vi "Panel.vi"(6 "Fiber Auto Collimation state data":refnum<class "Fiber Auto Collimation state data.lvclass">, 7 "Station config":refnum<class "Station config.lvclass">, 8 "error in":errorcluster, 11 "Fiber Auto Collimation main panel in":refnum<class "Fiber Auto Collimation main panel.lvclass">) -> (0 "error out":errorcluster, 3 "Fiber Auto Collimation main panel out":refnum<class "Fiber Auto Collimation main panel.lvclass">)   [LabVIEW 2018, in "Fiber Auto Collimation main panel.lvclass"]
doc: "The main panel of the station template when it's created. Adjust as needed!"
uses:
  Fiber Auto Collimation main panel.lvclass
  State data/BV Data.ctl
  C:/LabVIEW code/Fiber Auto Collimation/Source/Panels/Fiber Auto Collimation panel.lvclass
  State data/Fiber Auto Collimation state data.lvclass
  <userlib>/Recipe/Station Config/Station config.lvclass
  C:/Program Files (x86)/National Instruments/LabVIEW 2018/user.lib/Recipe/nLight Recipe/nLight Recipe.lvclass
  State data/Permission levels.ctl
  State data/Tracked state data.ctl
  State data/Instrument list.ctl
  State data/Fiber Auto Collimation state data.lvclass/Fiber Auto Collimation state data.ctl
  State data/String keys.ctl
  <userlib>/Recipe/Station Config/Station config.lvclass/Station config.ctl
  403c9101-8a94-4915-b1d2-c2bcb50c0ac3.vi
  4715e2b4-8d0b-45f9-9f48-fce3cbe10ad4.vi
  ee343da0-43c2-4897-a8b1-c706a9c51c79.vi
  88e119a9-a23e-4267-b647-8cd8f19a308b.vi
  457d34be-29b3-4e5e-81a2-a964ebca1608.vi
  94bc7fe1-a039-41b1-a3da-682790e1e5e6.vi
  5b4d40ab-973c-4ebc-87e6-d7e06bf2d1ec.vi
  373ea118-2318-4414-a1df-ab0a70bb7f1d.vi
  0939716d-f432-4146-8606-eb2c000bf93c.vi
  14963872-09c7-484d-8f8b-814a5689ce7f.vi
  226fbdc5-8833-4035-85a3-cb53d1a6b5a4.vi
  403c9101-8a94-4915-b1d2-c2bcb50c0ac3.vi/f33612d2-cbd2-4a12-8b29-77b7af87b990.vi
  88e119a9-a23e-4267-b647-8cd8f19a308b.vi/82f232c0-e180-498c-b36d-e812967a056b.vi
  References/Obtain control updates queue.vi
  Misc SubVIs/Get control name.vi
  <userlib>/nLight Error Handling/Merge errors no loss.vi
  <userlib>/nLight Error Handling/Replace string to enum conversion error.vi
  <userlib>/nLight Error Handling/Insert error no loss.vi
  <instrlib>/nLight Instruments/Monitor/Read History array.vi
  <vilib>/Utility/Data Type/Get Type Information.vi
  <userlib>/nLight Error Handling/Log any errors.vi
  <userlib>/Recipe/Test Recipe classes/Test Recipe.lvclass
  <instrlib>/nLight Instruments/nLight Instrument/nLight Instrument.lvclass
  <instrlib>/nLight Instruments/Monitor/Monitor.lvclass
  a23b397d-d5c1-4275-a046-494f1c6e56ee.vi
  <userlib>/Recipe/nLight Recipe/nLight Recipe.lvclass
  <userlib>/nEQdb/Test Data classes/Test Data.lvclass
  References/Fiber Auto Collimation References.lvclass
  Fiber Auto Collimation panel.lvclass
panel:
  in  "Defect detection":bool
  in  "Save Data":bool
  in  "SN selection":string(combo)
  in  "Step Size 6":bool
  in  "Step Size 5":bool
  in  "Step Size 4":bool
  in  "Step Size 3":bool
  in  "Step Size 2":bool
  in  "Step Size 1":bool
  in  "Spot detection":bool
  in  "Collimation":bool
  in  "Manual Mode":bool
  in  "Auto Mode":bool
  in  "Operator":string
  in  "Fiber Ass PN":string
  in  "SN-5":string
  in  "SN-4":string
  in  "SN-3":string
  in  "SN-2":string
  in  "SN-1":string
  in  "MOM Lot-2":string caption="MOM Lot"
  out "Measurement Report":string
  out "Collimation Image":T1(plugin-control)
  out "BV Data":T2={"Centroid X[um]"=nan, "Centroid Y[um]"=nan, "PeakResp.[%]"=nan, "Knife Edge X[mm]"=nan, "Knife Edge Y[mm]"=nan, "Circularity"=nan, "Collimation Result"=FALSE}
  in  "Cancel Test":bool
  in  "Start Test":bool
  in  "Enter MOM Lot":bool
  out "Test status":string
  out "MOM Lot":string
  out "Recipe Name":string
  out "Test in progress":bool
  out "DUT Serial":string
  out "Current Position[mm]":dbl
  in  "Home":bool
  in  "Down":bool
  in  "Up":bool
  out "Distance":dbl[unit] caption="Current step size" min=-0.001 max=0.025 step=0.001
  in  "Remote stop config panel":bool
  in  "Open and embed config panel":bool
  in  "Open config panel":bool
  out "Station information":string="Software name: \nSoftware version:\nSite: \nEnvironment: \nNEQdb Station number: \nMOM Equipment ID: "
  out "Monitored Watt indicator":dbl[unit]
  out "Fake LIV graph - Should be deleted later":T3(graph)
  out "Currently running state":string
  out "Username":string
  out "Permission level":T4
  out "Monitor Status":string
  # "INTRODUCE"
  # "Adjustment"
  # "Step size:"
  # "未连接MOM系统\n暂不使用"
  # "Settings"
  # "For the demo Monitor code.  Delete if not using Monitors at all.  If using Monitors, it may be useful to leave these as example code until after you implement your own monitors.  If so, you should probably hide both controls instead."
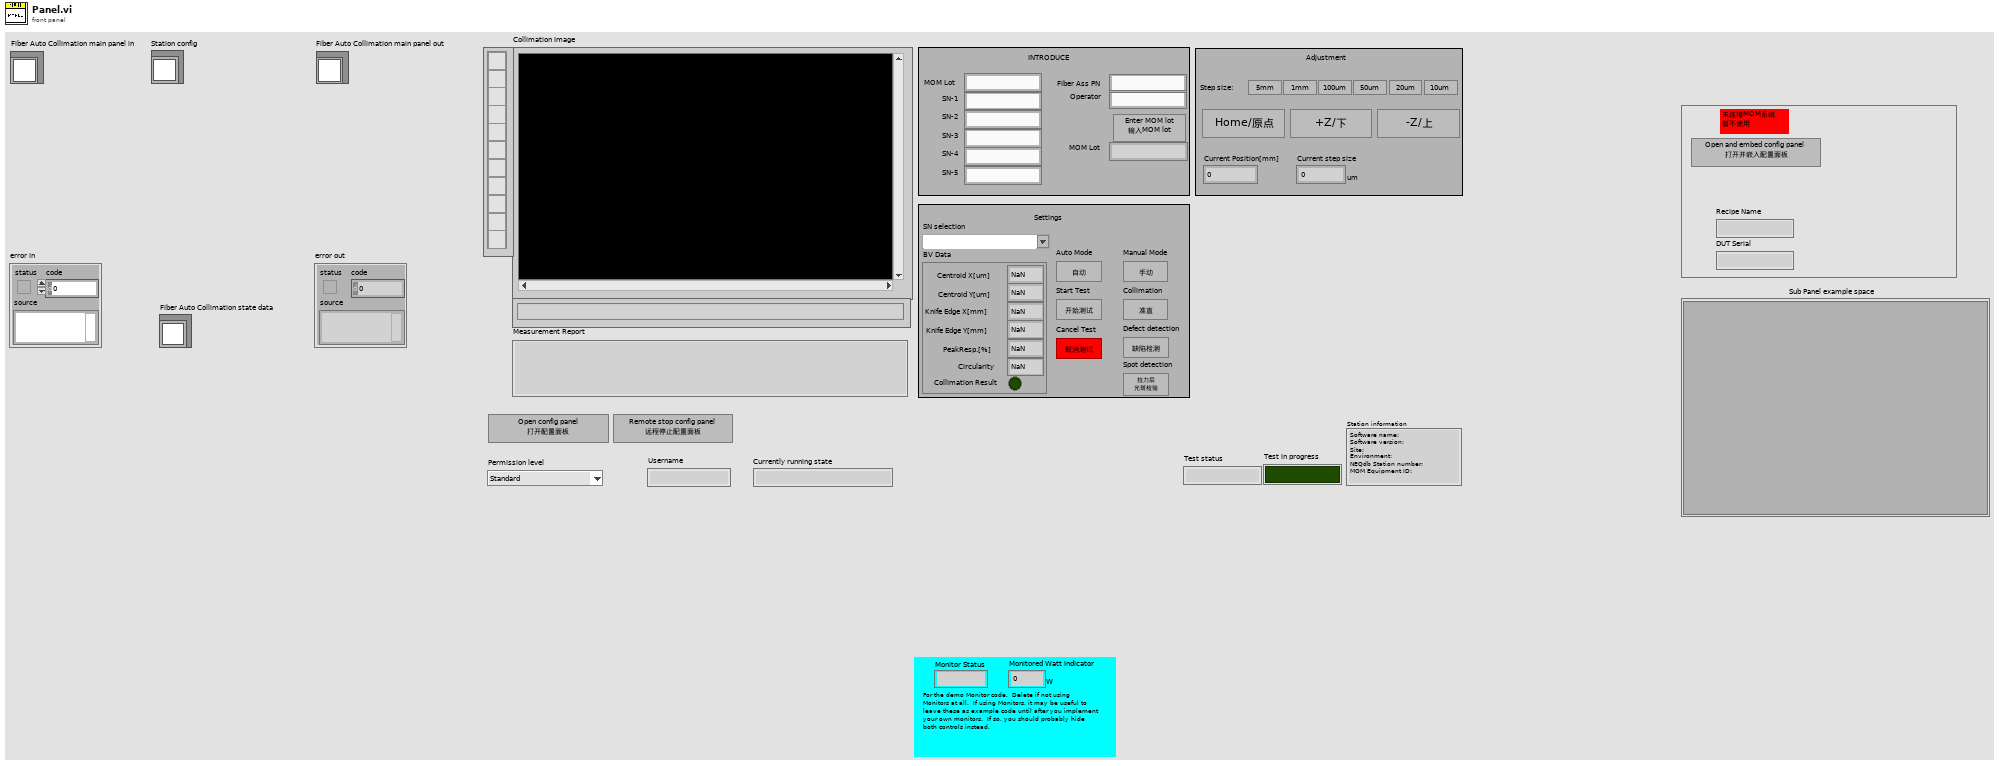
[diagram p1: front panel]
types:
  T1 = typedef "IMAQ Image.ctl" = refnum<image>
  T2 = typedef "Fiber Auto Collimation state data.lvclass/BV Data.ctl" = cluster{"Centroid X[um]":sgl, "Centroid Y[um]":sgl, "PeakResp.[%]":dbl, "Knife Edge X[mm]":sgl, "Knife Edge Y[mm]":sgl, "Circularity":sgl, "Collimation Result":bool}
  T3 = cluster{"Set current":sgl[unit], "Optical power":sgl[unit]}[]
  T4 = typedef "Fiber Auto Collimation state data.lvclass/Permission levels.ctl" = enum16{"Standard", "Technician", "Engineer"}
  T5 = typedef "Fiber Auto Collimation state data.lvclass/Tracked state data.ctl" = enum16{"No update", "Permission level", "Username", "Test running", "DUT Serial", "Test status", "MOM Lot", "Loaded test recipe", "Model case running", "Station status", "BV data", "Defect Identify data", "Axis Position data", "Fiber Ass PN", "Operator", "RunTime", "VBAI", "Steps Cycle Time"}
  T6 = enum8{"Enabled", "Disabled", "Disabled and Grayed Out"}
  T7 = cluster{"事件注册引用句柄":refnum<event-registration>, "事件注册引用句柄":refnum<event-registration>}
  T8 = typedef "Fiber Auto Collimation state data.lvclass/Instrument list.ctl" = enum16{""}
  T9 = typedef "Fiber Auto Collimation state data.lvclass/String keys.ctl" = enum16{"Software version", "Software name", "Collimation Steps Data Path", "Collimation Data Path", "Defect detection Image Path"}
  T10 = typedef "Monitor.lvclass/Basic monitor types.ctl" = enum16{"Error", "Status", "Other", "Waveform", "X-Y Graph", "Coordinates", "Count", "No units", "Watts", "Volts", "Amps", "Ohms", "Joules", "Coulombs", "Farads", "Temperature", "Wavelength", "Hertz", "Time", "Volume over time", "Speed", "Distance", "Area", "Angle", "Weight", "Pressure", "Percentage", "Discrete"}
  T11 = typedef "Station config.lvclass/Station site.ctl" = enum16{"Not set", "Vancouver", "Hillsboro", "Shanghai", "Lohja"}
  T12 = typedef "Station config.lvclass/Station environment.ctl" = enum16{"Not set", "Production", "Test", "Development"}
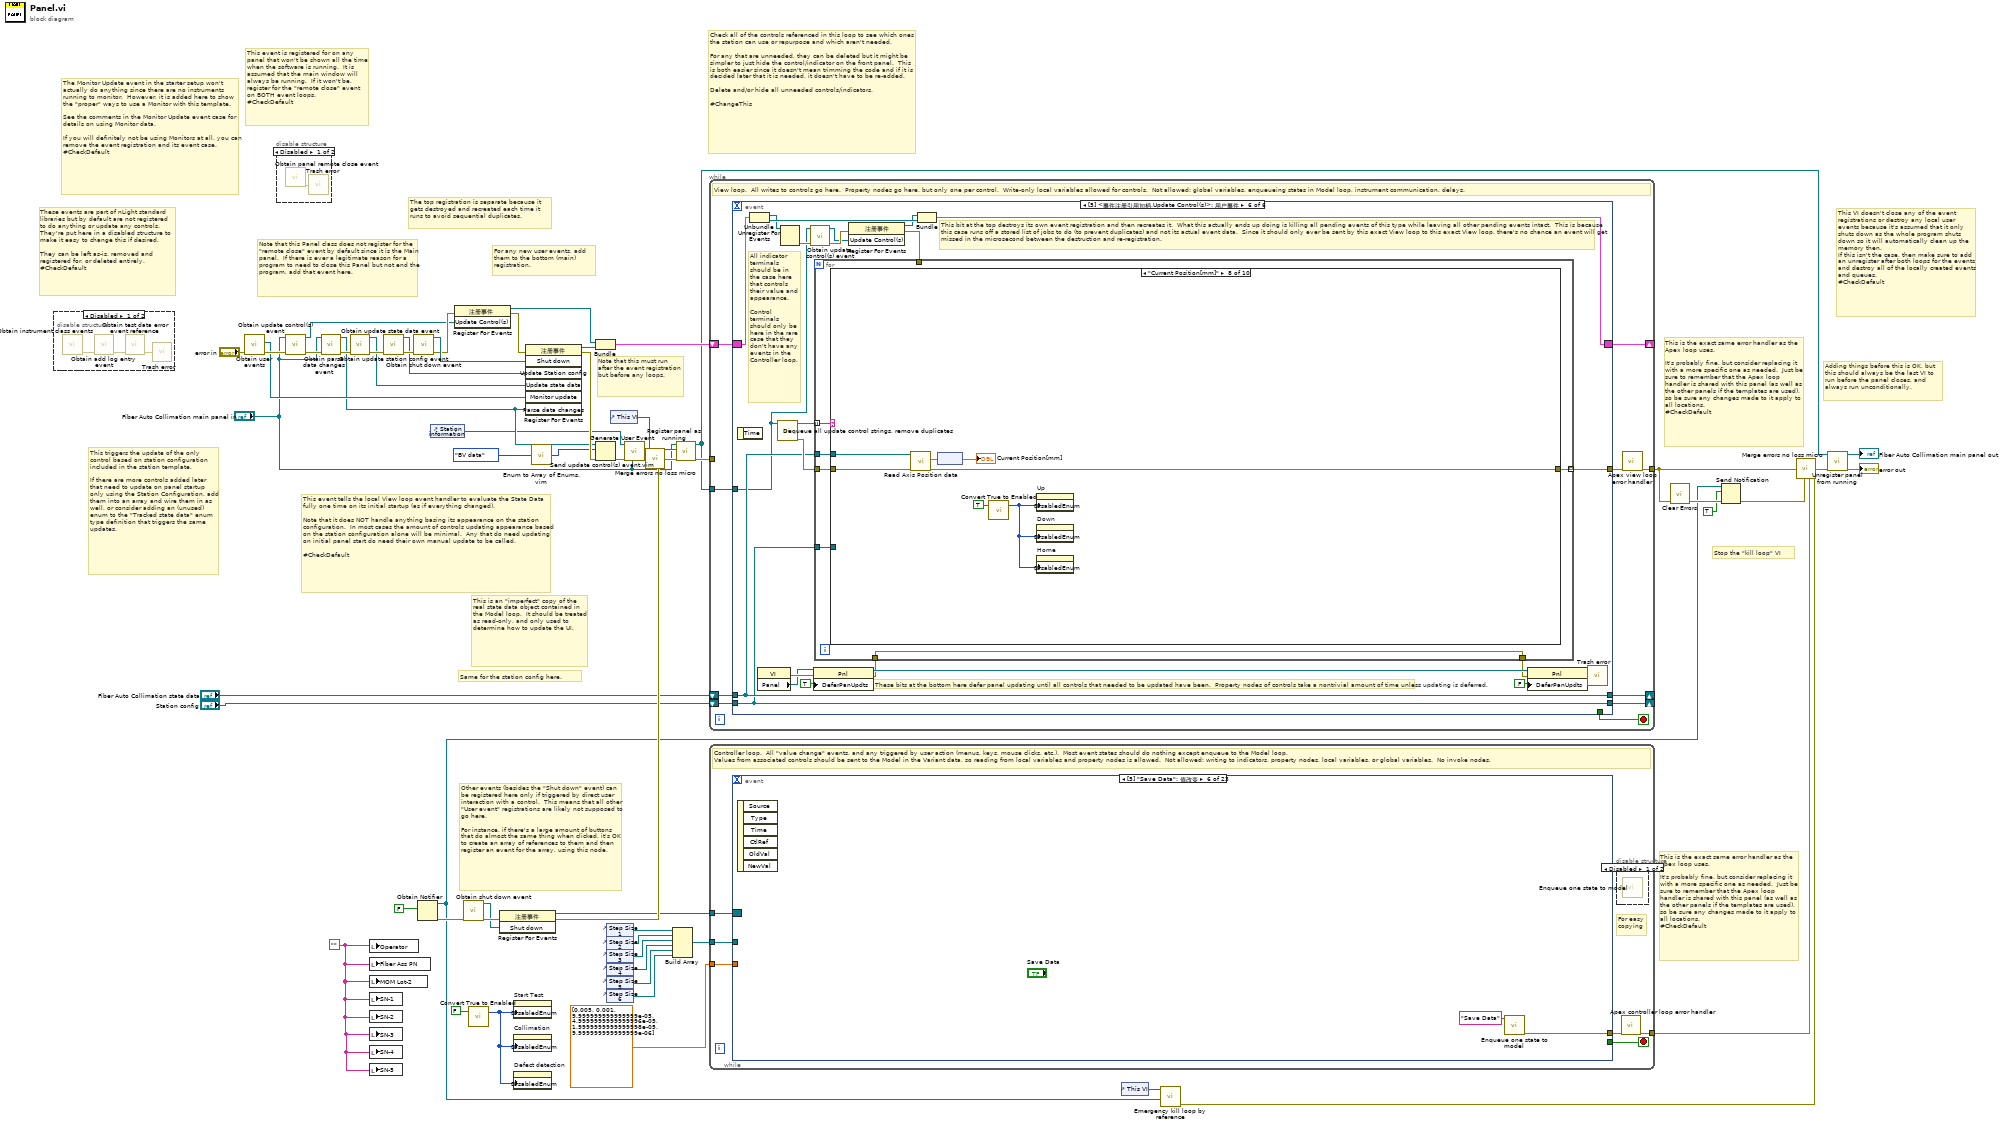
[diagram p0: block diagram]
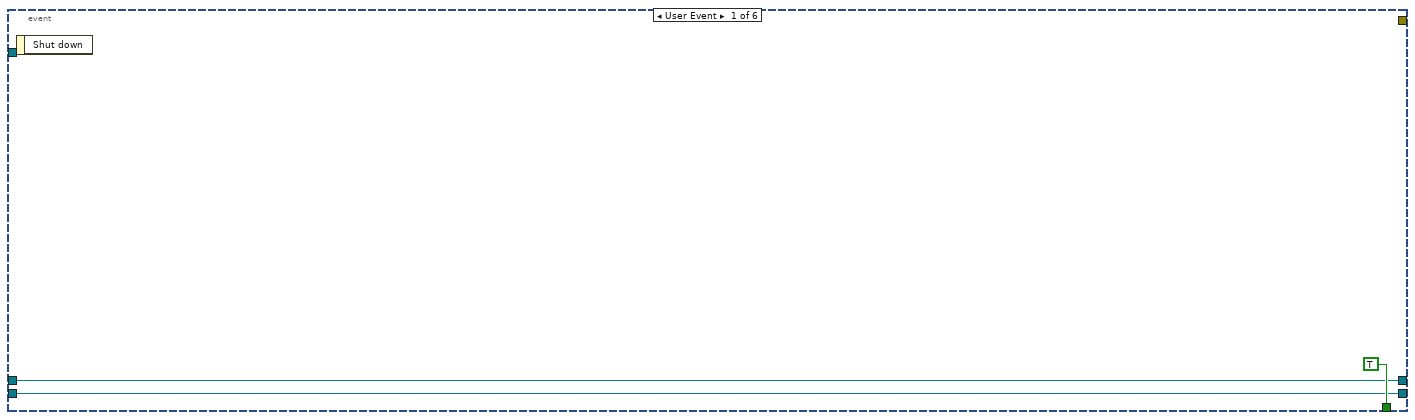
[diagram p4: hidden frame]
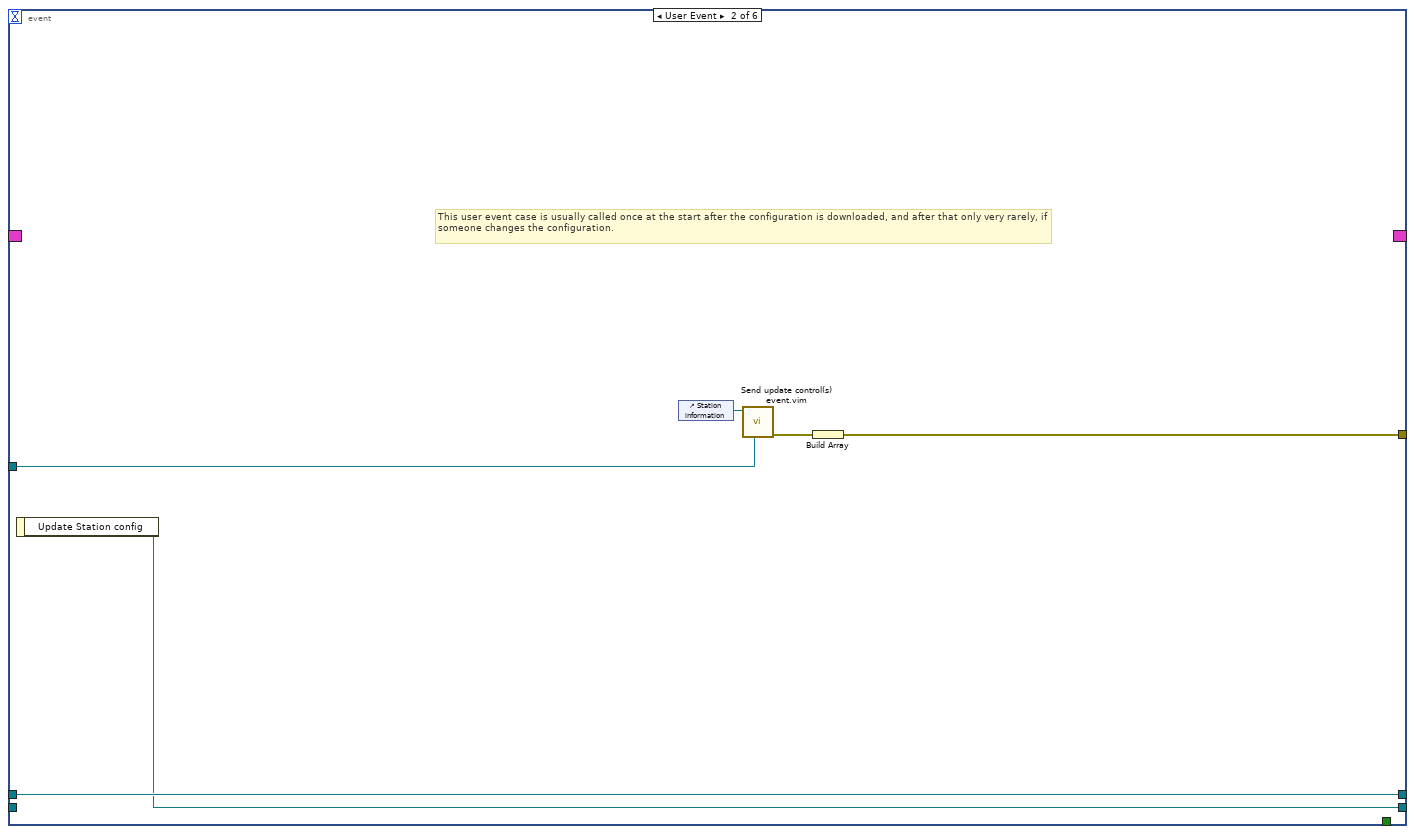
[diagram p5: hidden frame]
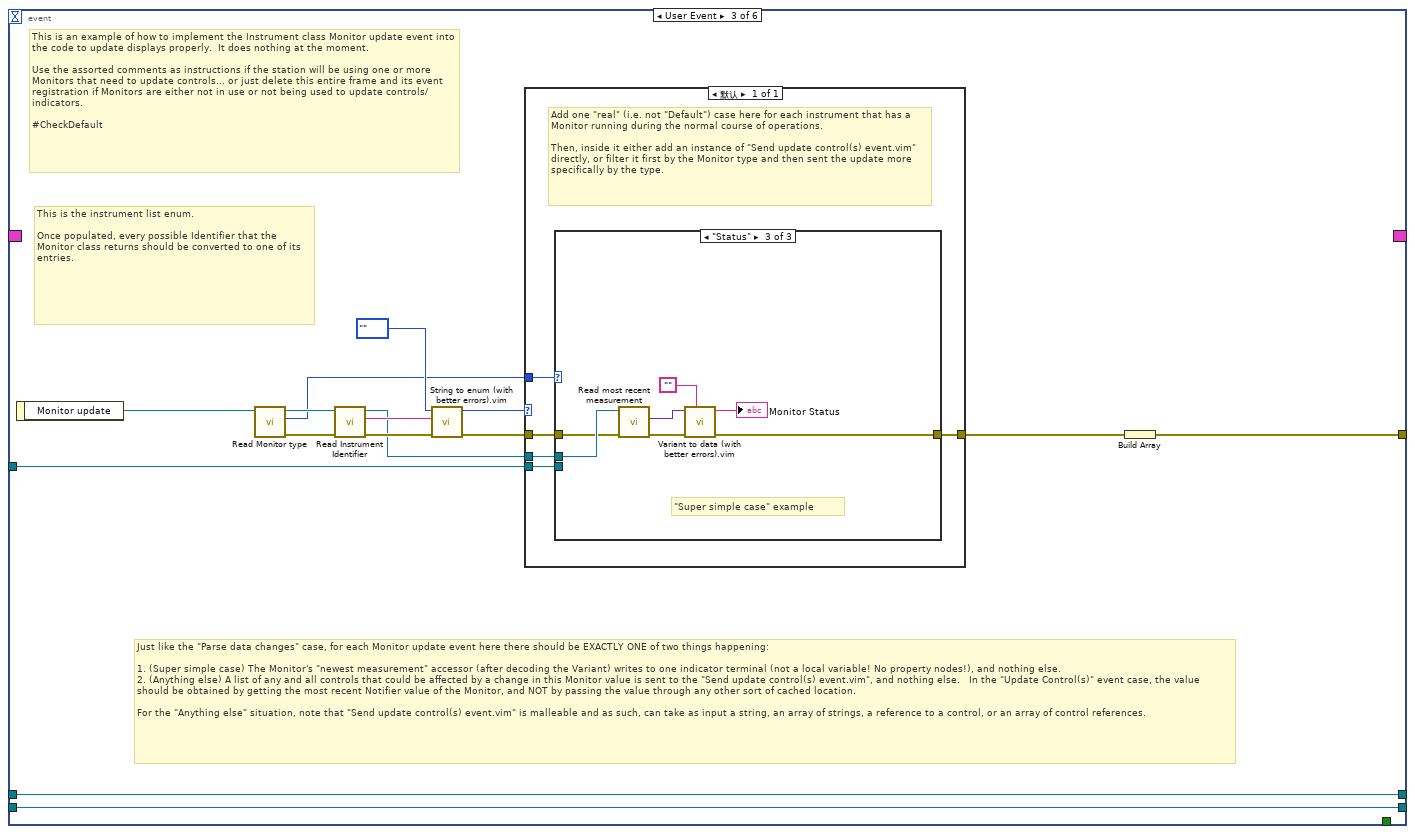
[diagram p6: hidden frame]
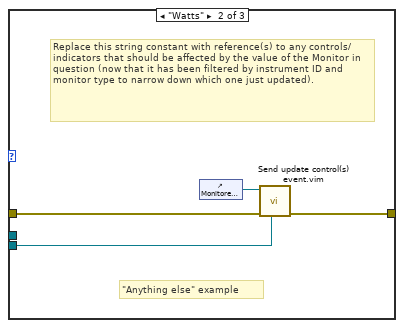
[diagram p8: hidden frame]
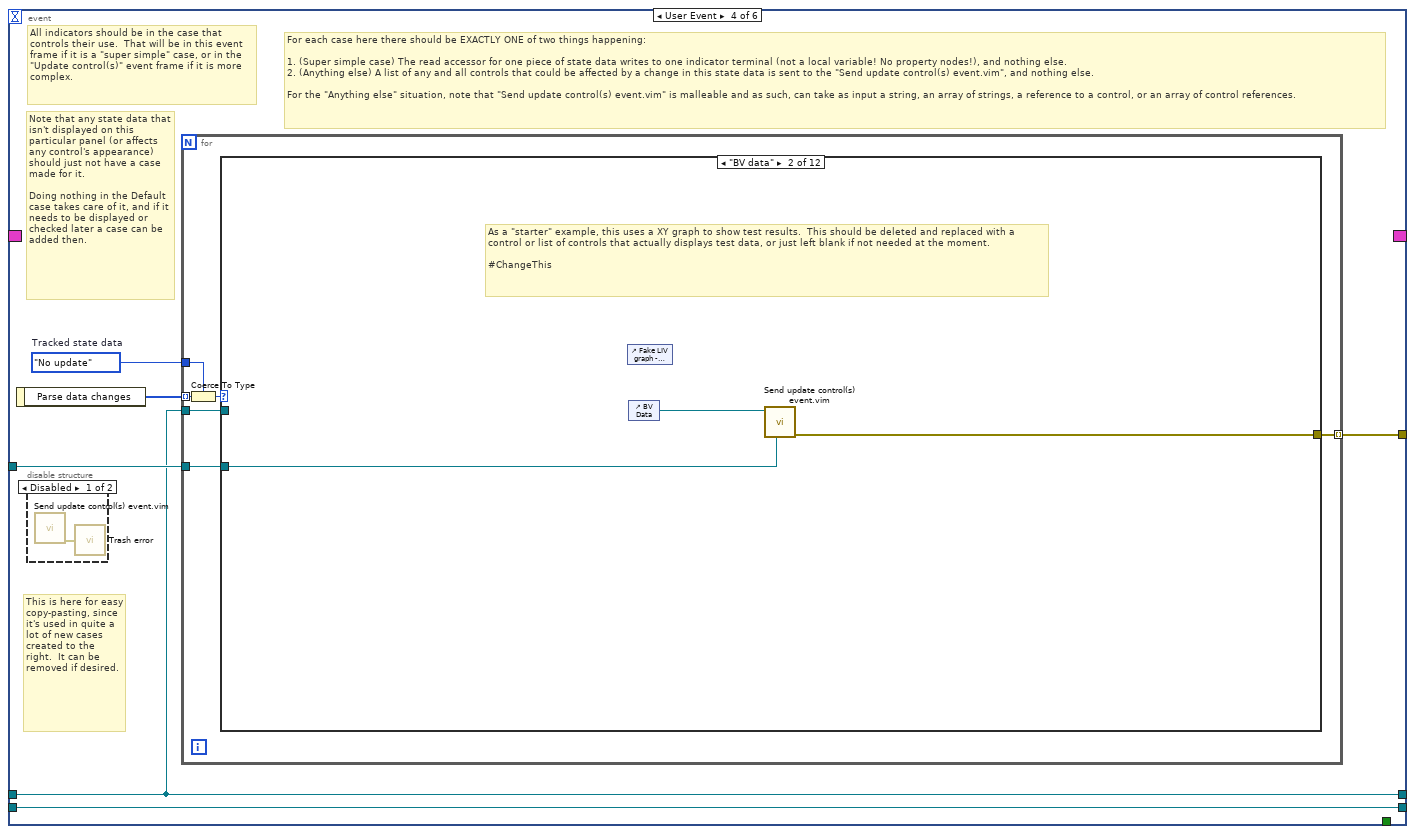
[diagram p9: hidden frame]
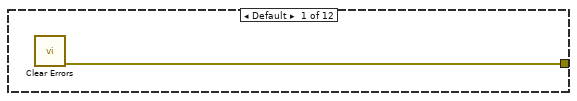
[diagram p11: hidden frame]
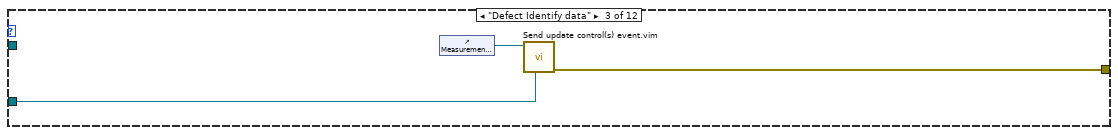
[diagram p12: hidden frame]
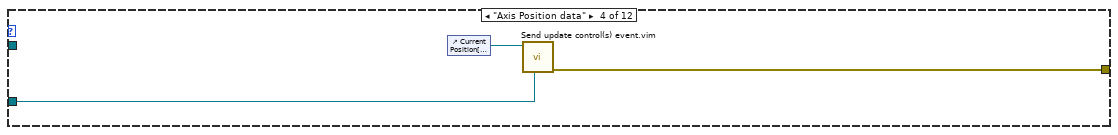
[diagram p13: hidden frame]
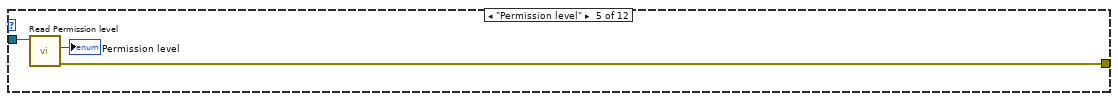
[diagram p14: hidden frame]
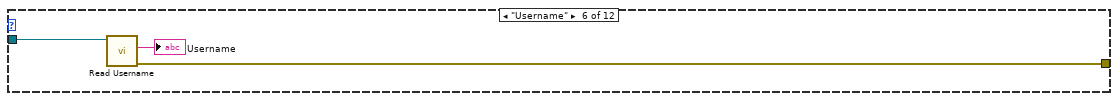
[diagram p15: hidden frame]
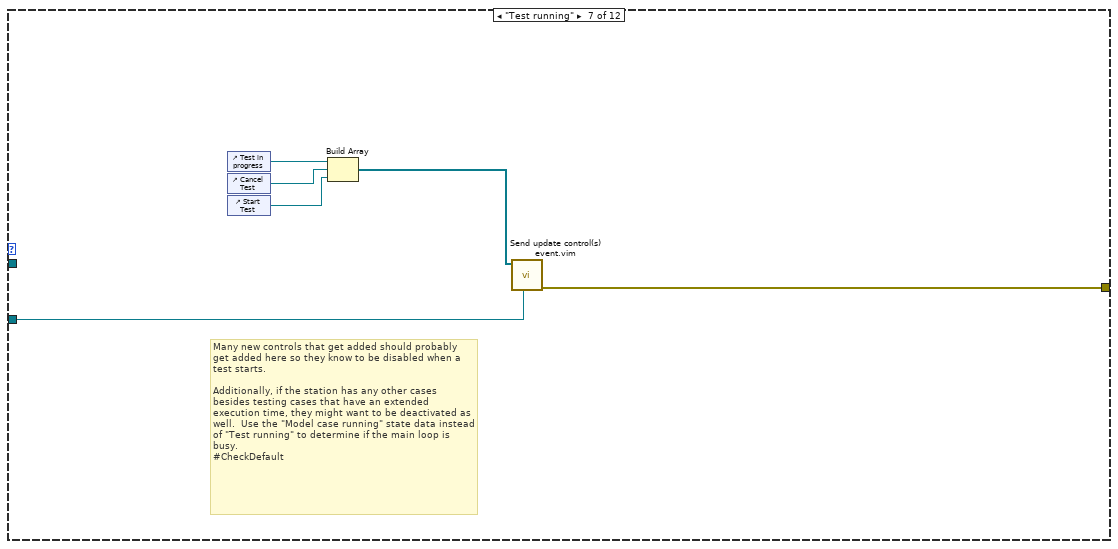
[diagram p16: hidden frame]
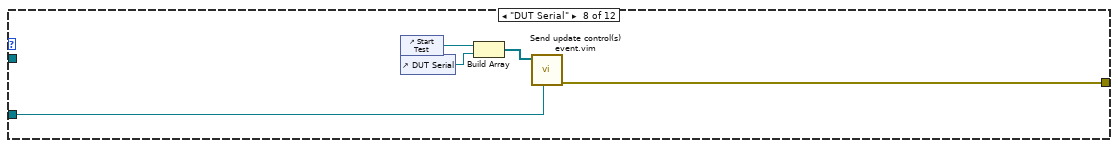
[diagram p17: hidden frame]
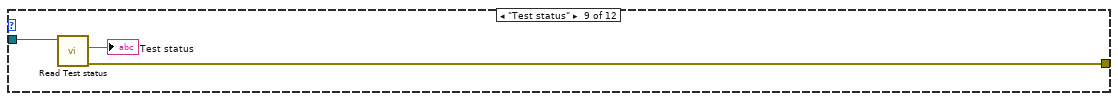
[diagram p18: hidden frame]
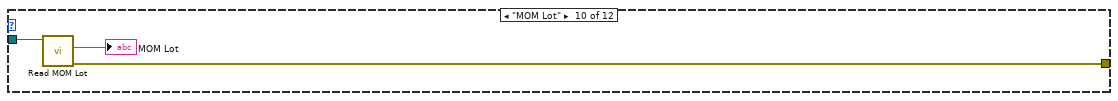
[diagram p19: hidden frame]
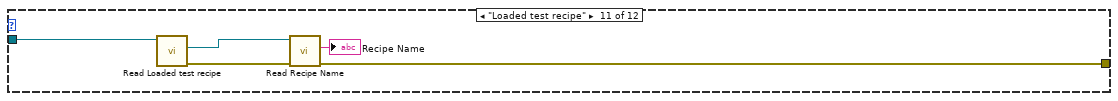
[diagram p20: hidden frame]
diagram:
  w1 = ""
  # "This VI doesn't close any of the event registrations or destroy any local user events because it's assumed that it only shuts down as the whole program shuts down so it will automatically clean up the memory then.\nIf this isn't the case, then make sure to add an unregister after both loops for the events and destroy all of the locally created events and queues.\n#CheckDefault"
  # "This event is registered for on any panel that won't be shown all the time when the software is running.  It is assumed that the main window will always be running.  If it won't be, register for the \"remote close\" event on BOTH event loops.\n#CheckDefault"
  # "Note that this Panel class does not register for the \"remote close\" event by default since it is the Main panel.  If there is ever a legitimate reason for a program to need to close this Panel but not end the program, add that event here."
  # "Note that this must run after the event registration but before any loops."
  # "This is the exact same error handler as the Apex loop uses.\n\nIt's probably fine, but consider replacing it with a more specific one as needed.  Just be sure to remember that the Apex loop handler is shared with this panel (as well as the other panels if the templates are used), so be sure any changes made to it apply to all locations.\n#CheckDefault"
  # "This is the exact same error handler as the Apex loop uses.\n\nIt's probably fine, but consider replacing it with a more specific one as needed.  Just be sure to remember that the Apex loop handler is shared with this panel (as well as the other panels if the templates are used), so be sure any changes made to it apply to all locations.\n#CheckDefault"
  # "This triggers the update of the only control based on station configuration included in the station template.\n\nIf there are more controls added later that need to update on panel startup only using the Station Configuration, add them into an array and wire them in as well, or consider adding an (unused) enum to the \"Tracked state data\" enum type definition that triggers the same updates."
  # "This event tells the local View loop event handler to evaluate the State Data fully one time on its initial startup (as if everything changed).\n\nNote that it does NOT handle anything basing its appearance on the station configuration.  In most cases the amount of controls updating appearance based on the station configuration alone will be minimal.  Any that do need updating on initial panel start do need their own manual update to be called.\n\n#CheckDefault"
  # "Adding things before this is OK, but this should always be the last VI to run before the panel closes, and always run unconditionally."
  # "Stop the \"kill loop\" VI"
  # "Same for the station config here."
  # "The Monitor Update event in the starter setup won't actually do anything since there are no instruments running to monitor.  However, it is added here to show the \"proper\" ways to use a Monitor with this template.  \n\nSee the comments in the Monitor Update event case for details on using Monitor data.\n\nIf you will definitely not be using Monitors at all, you can remove the event registration and its event case.\n#CheckDefault"
  # "Check all of the controls referenced in this loop to see which ones the station can use or repurpose and which aren't needed.  \n\nFor any that are unneeded, they can be deleted but it might be simpler to just hide the control/indicator on the front panel.  This is both easier since it doesn't mean trimming the code and if it is decided later that it is needed, it doesn't have to be re-added.\n\nDelete and/or hide all unneeded controls/indicators.\n\n#ChangeThis"
  # "Other events (besides the \"Shut down\" event) can be registered here only if triggered by direct user interaction with a control.  This means that all other \"User event\" registrations are likely not supposed to go here.\n\nFor instance, if there's a large amount of buttons that do almost the same thing when clicked, it's OK to create an array of references to them and then register an event for the array, using this node."
  # "For any new user events, add them to the bottom (main) registration."
  # "These events are part of nLight standard libraries but by default are not registered to do anything or update any controls.  They're put here in a disabled structure to make it easy to change this if desired.\n\nThey can be left as-is, removed and registered for, or deleted entirely.\n#CheckDefault"
  # "The top registration is separate because it gets destroyed and recreated each time it runs to avoid sequential duplicates."
  # "This is an \"imperfect\" copy of the real state data object contained in the Model loop.  It should be treated as read-only, and only used to determine how to update the UI."
  n1 = disable-structure shown="Disabled" {
    frame Disabled {
      n2 = call <instrlib>:"Obtain instrument class events.vi"() -> ("error out"=w61:errorcluster)  [unwired: 7 in, 4 out]
      n3 = call <userlib>:"Obtain add log entry event.vi"("error in (no error)"=w61) -> ("error out"=w60:errorcluster)  [unwired: 9 in, 1 out]
      n4 = call <userlib>:"Obtain test data error event reference.vi"("error in (no error)"=w60) -> ("error out"=w59:errorcluster)  [unwired: 9 in, 1 out]
      n5 = call <userlib>:"Trash error.vi"("error in"=w59) -> ()  [unwired: 15 in]
    }
    frame Enabled {
    }
  }
  n6 = call <instrlib>:"Obtain user events.vi"("error in (no error)"="error in") -> ("error out"=w42:errorcluster, "Monitor update"=w41:refnum<user-event>)  [unwired: 3 in, 6 out]
  n7 = disable-structure shown="Disabled" {
    frame Disabled {
      n8 = call "Obtain panel remote close event.vi"() -> ("error out"=w62:errorcluster)  [unwired: 10 in, 1 out]
      n9 = call <userlib>:"Trash error.vi"("error in"=w62) -> ()  [unwired: 15 in]
    }
    frame Enabled {
    }
  }
  n10 = call "Obtain update control(s) event.vi"("error in (no error)"=w42, "Fiber Auto Collimation panel"="Fiber Auto Collimation main panel in") -> ("error out"=w22:errorcluster, "Update Control(s)"=w44:refnum<user-event>)  [unwired: 8 in]
  n11 = call "Obtain parse data changes event.vi"("error in (no error)"=w22, "Fiber Auto Collimation panel"="Fiber Auto Collimation main panel in") -> ("error out"=w21:errorcluster, "Parse data changes"=w19:refnum<user-event>)  [unwired: 8 in]
  n12 = call "Obtain update state data event.vi"("error in (no error)"=w21) -> ("error out"=w54:errorcluster, "Update state data"=w47:refnum<user-event>)  [unwired: 9 in]
  n13 = local write "Operator"(w1) -> ()
  n14 = local write "Fiber Ass PN"(w1) -> ()
  n15 = local write "MOM Lot-2"(w1) -> ()
  n16 = local write "SN-1"(w1) -> ()
  n17 = local write "SN-2"(w1) -> ()
  n18 = local write "SN-3"(w1) -> ()
  n19 = local write "SN-4"(w1) -> ()
  n20 = local write "SN-5"(w1) -> ()
  n21 = call "Obtain update station config event.vi"("error in"=w54) -> ("error out"=w49:errorcluster, "Update Station config"=w48:refnum<user-event>)  [unwired: 9 in]
  n22 = call "Obtain shut down event.vi"("error in (no error)"=w49) -> ("error out"=w45:errorcluster, "Shut down"=w53:refnum<user-event>)  [unwired: 9 in]
  n23 = Obtain Notifier(notification data type=FALSE) -> (notifier out=w35:refnum<notifier>, error out=w38:errorcluster)  [unwired: 3 in, 1 out]
  n24 = control-ref of="Station information"() -> (w17:refnum<vi>)
  n25 = register-events(error in=w45, w44) -> (reference out=w43:refnum<event-registration>, error out=w28:errorcluster)  [unwired: 1 in]
  n26 = call "Obtain shut down event.vi"("error in (no error)"=w38) -> ("error out"=w52:errorcluster, "Shut down"=w51:refnum<user-event>)  [unwired: 9 in]
  n27 = call <userlib>:"Convert True to Enabled.vi"("Enable?"=FALSE) -> ("Enabled"=w3:T6)  [unwired: 2 in]
  n28 = register-events(error in=w52, w51) -> (reference out=w50:refnum<event-registration>, error out=w56:errorcluster)  [unwired: 1 in]
  n29 = property on="Start Test" class="Bool"("DisabledEnum"=w3) -> ()  [unwired: 2 in, 2 out]
  n30 = property on="Collimation" class="Bool"("DisabledEnum"=w3) -> ()  [unwired: 2 in, 2 out]
  n31 = property on="Defect detection" class="Bool"("DisabledEnum"=w3) -> ()  [unwired: 2 in, 2 out]
  n32 = register-events(error in=w28, w53, w48, w47, w41, w19) -> (reference out=w46:refnum<event-registration>, error out=w55:errorcluster)  [unwired: 1 in]
  n33 = call "Enum to Array of Enums.vim"("enum"=Tracked_state_data."BV data" ("Tracked state data")) -> ("array of enums"=w18:T5[])
  n34 = Bundle("事件注册引用句柄"=w43, "事件注册引用句柄"=w46) -> (w40:T7)  [unwired: 1 in]
  n35 = Generate User Event(user event=w19, event data cluster=w18, error in=w55) -> (error out=w16:errorcluster)  [unwired: 1 in, 1 out]
  n36 = control-ref of="Step Size 1"() -> (w11:refnum<vi>)
  n37 = control-ref of="Step Size 2"() -> (w10:refnum<vi>)
  n38 = control-ref of="Step Size 3"() -> (w9:refnum<vi>)
  n39 = control-ref of="Step Size 4"() -> (w8:refnum<vi>)
  n40 = control-ref of="Step Size 5"() -> (w7:refnum<vi>)
  n41 = control-ref of="Step Size 6"() -> (w6:refnum<vi>)
  n42 = control-ref of="This VI"() -> (w27:refnum<vi>)
  n43 = call "Send update control(s) event.vim"("Fiber Auto Collimation panel"="Fiber Auto Collimation main panel in", "error in"=w16, "Control(s) [String or reference, can be array]"=w17) -> ("error out"=w12:errorcluster)  [unwired: 8 in]
  n44 = call <userlib>:"Merge errors no loss micro.vi"("error in (no error) 1"=w12, "error in (no error) 6"=w56) -> ("error out"=w57:errorcluster)  [unwired: 7 in]
  n45 = Build Array(w11, w10, w9, w8, w7, w6) -> (w5:refnum<vi>[])
  n46 = call "Register panel as running.vi"("error in (no error)"=w57, "\"This VI\" reference from current panel"=w27, "Fiber Auto Collimation panel in"="Fiber Auto Collimation main panel in") -> ("error out"=w58:errorcluster, "Fiber Auto Collimation panel out"=w14:refnum<class "Fiber Auto Collimation main panel.lvclass">)  [unwired: 7 in]
  n47 = while {
    tunnel: [w72] -> w31
    shift-right: [w68] -> _
    shift-left: "Fiber Auto Collimation state data" -> [w67]
    shift-right: [w66] -> _
    shift-left: w40 -> [w71]
    shift-right: [w65] -> _
    shift-left: "Station config" -> [w64]
    tunnel: w14 -> [w63]
    tunnel: w58 -> [_]
    stop <- w69 stop-if-true
    # "View loop.  All writes to controls go here.  Property nodes go here, but only one per control.  Write-only local variables allowed for controls.  Not allowed: global variables, enqueueing states in Model loop, instrument communication, delays."
    n48 = event "View" shown="[5] <事件注册引用句柄.Update Control(s)>: 用户事件" {
      selector: w71 -> [_ _ _ _ _ w199]
      dyn-events: [_ _ _ _ _ w192] -> w66
      timeout: _ -> [_ _ _ _ _ _]
      tunnel: [_ w77 w85 w119 w173 w181] -> w70
      tunnel: [TRUE _ _ _ _ _] -> w69
      tunnel: [w74 w81 w96 w116 w170 w182] -> w68
      tunnel: w67 -> [w74 w81 w96 w116 _ w182]
      tunnel: [w73 w80 w84 w118 w176 w179] -> w65
      tunnel: w64 -> [w73 _ w84 w118 w176 w179]
      tunnel: w63 -> [_ w76 w82 w117 w175 w178]
      event User Event {
        n49 = event-data() -> ()  [unwired: 1 in, 1 out]
      }
      event User Event {
        # "This user event case is usually called once at the start after the configuration is downloaded, and after that only very rarely, if someone changes the configuration."
        n50 = event-data() -> ("Update Station config"=w80:refnum<class "Station config.lvclass">)  [unwired: 1 in]
        n51 = control-ref of="Station information"() -> (w79:refnum<vi>)
        n52 = call "Send update control(s) event.vim"("Fiber Auto Collimation panel"=w76, "Control(s) [String or reference, can be array]"=w79) -> ("error out"=w78:errorcluster)  [unwired: 9 in]
        n53 = Build Array(w78) -> (w77:errorcluster[])
      }
      event User Event {
        # "Just like the \"Parse data changes\" case, for each Monitor update event here there should be EXACTLY ONE of two things happening:\n\n1. (Super simple case) The Monitor's \"newest measurement\" accessor (after decoding the Variant) writes to one indicator terminal (not a local variable! No property nodes!), and nothing else.\n2. (Anything else) A list of any and all controls that could be affected by a change in this Monitor value is sent to the \"Send update control(s) event.vim\", and nothing else.   In the \"Update Control(s)\" event case, the value should be obtained by getting the most recent Notifier value of the Monitor, and NOT by passing the value through any other sort of cached location.\n\nFor the \"Anything else\" situation, note that \"Send update control(s) event.vim\" is malleable and as such, can take as input a string, an array of strings, a reference to a control, or an array of control references."
        # "This is the instrument list enum.\n\nOnce populated, every possible Identifier that the Monitor class returns should be converted to one of its entries."
        # "This is an example of how to implement the Instrument class Monitor update event into the code to update displays properly.  It does nothing at the moment.  \n\nUse the assorted comments as instructions if the station will be using one or more Monitors that need to update controls... or just delete this entire frame and its event registration if Monitors are either not in use or not being used to update controls/indicators.\n\n#CheckDefault"
        n54 = event-data() -> ("Monitor update"=w95:refnum<class "Monitor.lvclass">)  [unwired: 1 in]
        n55 = call <instrlib>:"Read Monitor type.vi"("Monitor in"=w95) -> ("error out"=w93:errorcluster, "Basic monitor types"=w87:T10, "Monitor out"=w94:refnum<class "Monitor.lvclass">)  [unwired: 8 in]
        n56 = call <instrlib>:"Read Instrument Identifier.vi"("error in (no error)"=w93, "Monitor in"=w94) -> ("error out"=w92:errorcluster, "Instrument Identifier"=w90:string, "Monitor out"=w83:refnum<class "Monitor.lvclass">)  [unwired: 7 in]
        n57 = call "String to enum (with better errors).vim"("error in (no error)"=w92, "Text to be converted"=w90, "Default enum value"=Instrument_list."" ("Instrument list")) -> ("error out"=w88:errorcluster, "Converted value out"=w89:T8)  [unwired: 7 in]
        n58 = case shown="默认" w89 {
          tunnel: w88 -> [w101]
          tunnel: w87 -> [w100]
          tunnel: [w99] -> w86
          tunnel: w83 -> [w98]
          tunnel: w82 -> [w97]
          frame 默认 {
            # "Add one \"real\" (i.e. not \"Default\") case here for each instrument that has a Monitor running during the normal course of operations.\n\nThen, inside it either add an instance of \"Send update control(s) event.vim\" directly, or filter it first by the Monitor type and then sent the update more specifically by the type."
            n59 = case shown="\"Status\"" w100 {
              tunnel: w101 -> [w102 w106 w112]
              tunnel: [w102 w105 w107] -> w99
              tunnel: w98 -> [_ _ w113]
              tunnel: w97 -> [_ w103 _]
              frame Default {
                # "Default case probably shouldn't be used to send control updates.  \n\nPossibly add an error generator here, though... it will generate errors to \"remind\" you that if you add a Monitor elsewhere, you need to add a case for it here."
              }
              frame "Watts" {
                # "\"Anything else\" example"
                # "Replace this string constant with reference(s) to any controls/indicators that should be affected by the value of the Monitor in question (now that it has been filtered by instrument ID and monitor type to narrow down which one just updated)."
                n60 = control-ref of="Monitored Watt indicator"() -> (w104:refnum<vi>)
                n61 = call "Send update control(s) event.vim"("Fiber Auto Collimation panel"=w103, "error in"=w106, "Control(s) [String or reference, can be array]"=w104) -> ("error out"=w105:errorcluster)  [unwired: 8 in]
              }
              frame "Status" {
                # "\"Super simple case\" example"
                n62 = call <instrlib>:"Read most recent measurement.vi"("error in (no error)"=w112, "Monitor in"=w113) -> ("error out"=w111:errorcluster, "Latest value monitored"=w110:variant)  [unwired: 6 in, 2 out]
                n63 = call "Variant to data (with better errors).vim"("type"="", "error in"=w111, "variant"=w110) -> ("error out"=w107:errorcluster, "data"=→"Monitor Status":string)  [unwired: 7 in]
              }
            }
          }
        }
        n64 = Build Array(w86) -> (w85:errorcluster[])
      }
      event User Event {
        w114 = Tracked_state_data."No update"  # Tracked state data
        # "Note that any state data that isn't displayed on this particular panel (or affects any control's appearance) should just not have a case made for it.  \n\nDoing nothing in the Default case takes care of it, and if it needs to be displayed or checked later a case can be added then."
        # "All indicators should be in the case that controls their use.  That will be in this event frame if it is a \"super simple\" case, or in the \"Update control(s)\" event frame if it is more complex."
        # "This is here for easy copy-pasting, since it's used in quite a lot of new cases created to the right.  It can be removed if desired."
        # "For each case here there should be EXACTLY ONE of two things happening:\n\n1. (Super simple case) The read accessor for one piece of state data writes to one indicator terminal (not a local variable! No property nodes!), and nothing else.\n2. (Anything else) A list of any and all controls that could be affected by a change in this state data is sent to the \"Send update control(s) event.vim\", and nothing else.\n\nFor the \"Anything else\" situation, note that \"Send update control(s) event.vim\" is malleable and as such, can take as input a string, an array of strings, a reference to a control, or an array of control references."
        n65 = event-data() -> ("Parse data changes"=w115:u16[])  [unwired: 1 in]
        n66 = disable-structure shown="Disabled" {
          frame Disabled {
            n67 = call "Send update control(s) event.vim"() -> ("error out"=w120:errorcluster)  [unwired: 11 in]
            n68 = call <userlib>:"Trash error.vi"("error in"=w120) -> ()  [unwired: 15 in]
          }
          frame Enabled {
          }
        }
        n69 = for {
          tunnel: w115 -> [w126] mode=indexing
          tunnel: w116 -> [w125]
          tunnel: [w124] -> w119 mode=indexing
          tunnel: w117 -> [w123]
          tunnel: w114 -> [w121]
          n70 = Coerce To Type(0:w126, 1:w121) -> (2:w122:T5)
          n71 = case shown="\"BV data\"" w122 {
            tunnel: w125 -> [_ _ _ _ w139 w140 _ _ w156 w159 w164 w167]
            tunnel: [w127 w130 w132 w135 w138 w142 w148 w153 w155 w157 w160 w165] -> w124
            tunnel: w123 -> [_ w129 w133 w136 _ _ w143 w149 _ _ _ _]
            frame Default {
              n72 = call <vilib>:"Clear Errors.vi"() -> ("error out"=w127:errorcluster)  [unwired: 6 in, 1 out]
            }
            frame "BV data" {
              # "As a \"starter\" example, this uses a XY graph to show test results.  This should be deleted and replaced with a control or list of controls that actually displays test data, or just left blank if not needed at the moment.\n\n#ChangeThis"
              n73 = control-ref of="Fake LIV graph - Should be deleted later"() -> ()  [unwired: 1 out]
              n74 = control-ref of="BV Data"() -> (w128:refnum<vi>)
              n75 = call "Send update control(s) event.vim"("Fiber Auto Collimation panel"=w129, "Control(s) [String or reference, can be array]"=w128) -> ("error out"=w130:errorcluster)  [unwired: 9 in]
            }
            frame "Defect Identify data" {
              n76 = control-ref of="Measurement Report"() -> (w131:refnum<vi>)
              n77 = call "Send update control(s) event.vim"("Fiber Auto Collimation panel"=w133, "Control(s) [String or reference, can be array]"=w131) -> ("error out"=w132:errorcluster)  [unwired: 9 in]
            }
            frame "Axis Position data" {
              n78 = control-ref of="Current Position[mm]"() -> (w134:refnum<vi>)
              n79 = call "Send update control(s) event.vim"("Fiber Auto Collimation panel"=w136, "Control(s) [String or reference, can be array]"=w134) -> ("error out"=w135:errorcluster)  [unwired: 9 in]
            }
            frame "Permission level" {
              n80 = call "Read Permission level.vi"("Fiber Auto Collimation state data in"=w139) -> ("error out"=w138:errorcluster, "Permission level"=→"Permission level":T4)  [unwired: 8 in, 1 out]
            }
            frame "Username" {
              n81 = call "Read Username.vi"("Fiber Auto Collimation state data in"=w140) -> ("error out"=w142:errorcluster, "Username"=→"Username":string)  [unwired: 8 in, 1 out]
            }
            frame "Test running" {
              # "Many new controls that get added should probably get added here so they know to be disabled when a test starts.\n\nAdditionally, if the station has any other cases besides testing cases that have an extended execution time, they might want to be deactivated as well.  Use the \"Model case running\" state data instead of \"Test running\" to determine if the main loop is busy.\n#CheckDefault"
              n82 = control-ref of="Test in progress"() -> (w147:refnum<vi>)
              n83 = control-ref of="Cancel Test"() -> (w146:refnum<vi>)
              n84 = control-ref of="Start Test"() -> (w145:refnum<vi>)
              n85 = Build Array(w147, w146, w145) -> (w144:refnum<vi>[])
              n86 = call "Send update control(s) event.vim"("Fiber Auto Collimation panel"=w143, "Control(s) [String or reference, can be array]"=w144) -> ("error out"=w148:errorcluster)  [unwired: 9 in]
            }
            frame "DUT Serial" {
              n87 = control-ref of="Start Test"() -> (w152:refnum<vi>)
              n88 = control-ref of="DUT Serial"() -> (w151:refnum<vi>)
              n89 = Build Array(w152, w151) -> (w150:refnum<vi>[])
              n90 = call "Send update control(s) event.vim"("Fiber Auto Collimation panel"=w149, "Control(s) [String or reference, can be array]"=w150) -> ("error out"=w153:errorcluster)  [unwired: 9 in]
            }
            frame "Test status" {
              n91 = call "Read Test status.vi"("Fiber Auto Collimation state data in"=w156) -> ("error out"=w155:errorcluster, "Test status"=→"Test status":string)  [unwired: 8 in, 1 out]
            }
            frame "MOM Lot" {
              n92 = call "Read MOM Lot.vi"("Fiber Auto Collimation state data in"=w159) -> ("error out"=w157:errorcluster, "MOM Lot"=→"MOM Lot":string)  [unwired: 8 in, 1 out]
            }
            frame "Loaded test recipe" {
              n93 = call "Read Loaded test recipe.vi"("Fiber Auto Collimation state data in"=w164) -> ("error out"=w162:errorcluster, "Loaded test recipe"=w163:refnum<class "Test Recipe.lvclass">)  [unwired: 8 in, 1 out]
              n94 = call-dynamic "Read Recipe Name.vi"("error in (no error)"=w162, "nLight Recipe in"=w163) -> ("error out"=w160:errorcluster, "Recipe Name"=→"Recipe Name":string)  [unwired: 7 in, 1 out]
            }
            frame "Model case running" {
              n95 = call "Read Model case running.vi"("Fiber Auto Collimation state data in"=w167) -> ("error out"=w165:errorcluster, "Model case running"=→"Currently running state":string)  [unwired: 6 in, 3 out]
            }
          }
        }
      }
      event User Event {
        # "This case does two things:\n\n* Writes the new copy of the state data to the shift register\n* Sends out the \"Parse data changes\" event specific to this panel\n\nThis is an extra \"layer\" between the changing of state data and the changing of control appearance that does not exist on the main VI.  It is here so that when this Panel launches, it can internally trigger an update of all possible controls on itself that does not send a state data update event containing all possible items to all running panels at once."
        n96 = event-data() -> ("Update state data"=w170:refnum<class "Fiber Auto Collimation state data.lvclass">)  [unwired: 1 in]
        n97 = call "Read Changed data list.vi"("Fiber Auto Collimation state data in"=w170) -> ("error out"=w169:errorcluster, "Changed data list"=w168:T5[])  [unwired: 8 in, 1 out]
        n98 = call "Obtain parse data changes event.vi"("error in (no error)"=w169, "Fiber Auto Collimation panel"=w175) -> ("error out"=w174:errorcluster, "Parse data changes"=w171:refnum<user-event>)  [unwired: 8 in]
        n99 = Generate User Event(user event=w171, event data cluster=w168, error in=w174) -> (error out=w172:errorcluster)  [unwired: 1 in, 1 out]
        n100 = Build Array(w172) -> (w173:errorcluster[])
      }
      event User Event {
        # "All indicator terminals should be in the case here that controls their value and appearance.\n\nControl terminals should only be here in the rare case that they don't have any events in the Controller loop."
        # "These bits at the bottom here defer panel updating until all controls that needed to be updated have been.  Property nodes of controls take a nontrivial amount of time unless updating is deferred."
        # "This bit at the top destroys its own event registration and then recreates it.  What this actually ends up doing is killing all pending events of this type while leaving all other pending events intact.  This is because this case runs off a stored list of jobs to do (to prevent duplicates) and not its actual event data.  Since it should only ever be sent by this exact View loop to this exact View loop, there's no chance an event will get missed in the microsecond between the destruction and re-registration."
        n101 = event-data() -> ()  [unwired: 1 in, 1 out]
        n102 = Unbundle(w199) -> ("事件注册引用句柄"=w197:refnum<event-registration>, "事件注册引用句柄"=w198:refnum<event-registration>)
        n103 = property class="VI"() -> (error out=w191:errorcluster, "Panel"=w189:refnum<vi>)  [unwired: 2 in, 1 out]
        n104 = call "Dequeue all update control strings, remove duplicates.vi"("Fiber Auto Collimation panel"=w178) -> ("error out"=w186:errorcluster, "Controls to update"=w185:string[])  [unwired: 9 in]
        n105 = Unregister For Events(event registration refnum=w197) -> (error out=w196:errorcluster)  [unwired: 1 in]
        n106 = call "Obtain update control(s) event.vi"("error in (no error)"=w196, "Fiber Auto Collimation panel"=w178) -> ("error out"=w195:errorcluster, "Update Control(s)"=w194:refnum<user-event>)  [unwired: 8 in]
        n107 = property class="Pnl"(reference=w189, error in=w191, "DeferPanUpdts"=TRUE ("Defer Panel Updates")) -> (reference out=w187:refnum<vi>, error out=w184:errorcluster)
        n108 = register-events(error in=w195, w194) -> (reference out=w193:refnum<event-registration>, error out=w180:errorcluster)  [unwired: 1 in]
        n109 = for {
          tunnel: w186 -> [w204]
          tunnel: w185 -> [w205] mode=indexing
          tunnel: [w203] -> w181 mode=indexing
          tunnel: w184 -> [w202]
          tunnel: [w202] -> w183
          tunnel: w182 -> [w201]
          tunnel: w180 -> [_]
          tunnel: w179 -> [w200]
          n110 = case shown="\"Current Position[mm]\"" w205 {
            selector: w205 -> [w208 _ _ _ _ _ _ _ _ _]
            tunnel: w204 -> [w207 w221 w230 w234 w237 w242 w248 w255 w265 w269]
            tunnel: [w206 w218 w225 w231 w235 w240 w246 w251 w256 w266] -> w203
            tunnel: w201 -> [_ w220 w229 w233 w236 w241 w247 w254 _ _]
            tunnel: w200 -> [_ _ _ _ _ _ _ _ _ w268]
            frame Default {
              n111 = Format Into String(format string="Default case reached in \"Update control(s)\" event!\nIntended control name was \"%s\".", w208) -> (resulting string=w209:string)  [unwired: 2 in, 1 out]
              n112 = call <userlib>:"Insert impossible case error.vi"("error in (no error)"=w207, "Optional extra info"=w209) -> ("error out"=w206:errorcluster)  [unwired: 9 in]
            }
            frame "Start Test" {
              n113 = call "Read Test running.vi"("error in (no error)"=w221, "Fiber Auto Collimation state data in"=w220) -> ("error out"=w217:errorcluster, "Test running"=w215:bool, "Fiber Auto Collimation state data out"=w216:refnum<class "Fiber Auto Collimation state data.lvclass">)  [unwired: 6 in, 1 out]
              n114 = call "Read DUT Serial.vi"("error in (no error)"=w217, "Fiber Auto Collimation state data in"=w216) -> ("error out"=w211:errorcluster, "DUT Serial"=w214:string)  [unwired: 7 in, 1 out]
              n115 = disable-structure shown="禁用" {
                disable-tunnel: w214 -> [w223 _]
                disable-tunnel: [w222 FALSE] -> w213
                frame Enabled {
                  n116 = Empty String/Path?(string/path=w223) -> (empty?=w222:bool)
                }
                frame Disabled {
                  # "RCX"
                }
              }
              n117 = Not Or(1:w215, 2:w213) -> (0:w212:bool)
              n118 = call <userlib>:"Convert True to Enabled.vi"("Enable?"=w212) -> ("Enabled"=w219:T6)  [unwired: 2 in]
              n119 = property on="Start Test" class="Bool"(error in=w211, "DisabledEnum"=w219) -> (error out=w218:errorcluster)  [unwired: 1 in, 1 out]
            }
            frame "Cancel Test" {
              n120 = call "Read Test running.vi"("error in (no error)"=w230, "Fiber Auto Collimation state data in"=w229) -> ("error out"=w226:errorcluster, "Test running"=w228:bool)  [unwired: 6 in, 2 out]
              n121 = call <userlib>:"Convert True to Enabled.vi"("Enable?"=w228) -> ("Enabled"=w227:T6)  [unwired: 2 in]
              n122 = property on="Cancel Test" class="Bool"(error in=w226, "DisabledEnum"=w227) -> (error out=w225:errorcluster)  [unwired: 1 in, 1 out]
            }
            frame "Test in progress" {
              n123 = call "Read Test running.vi"("error in (no error)"=w234, "Fiber Auto Collimation state data in"=w233) -> ("error out"=w231:errorcluster, "Test running"=→"Test in progress":bool)  [unwired: 6 in, 2 out]
            }
            frame "DUT Serial" {
              n124 = call "Read DUT Serial.vi"("error in (no error)"=w237, "Fiber Auto Collimation state data in"=w236) -> ("error out"=w235:errorcluster, "DUT Serial"=→"DUT Serial":string)  [unwired: 7 in, 1 out]
            }
            frame "BV Data" {
              # "The graph here just uses autoscale to always show all the data.\n\nA \"real\" test data graph would probably be more intelligent, such as setting the outer bound to the last point in the test so the entire amp set point scale would be shown from the start, overlaying an efficiency rating or other data points, etc."
              # "So that if a lower current is added later, the graph still shows points in order"
              n125 = call "Read Collimation data.vi"("error in (no error)"=w242, "Fiber Auto Collimation state data in"=w241) -> ("error out"=w240:errorcluster, "BV Data"=→"BV Data":T2)  [unwired: 7 in, 1 out]
            }
            frame "Measurement Report" {
              n126 = call "Read Defect Identify data.vi"("error in (no error)"=w248, "Fiber Auto Collimation state data in"=w247) -> ("error out"=w246:errorcluster, "Defect Identify data"=w245:cluster{"Image":T1, "Measure Report":string})  [unwired: 7 in, 1 out]
              n127 = Unbundle By Name(w245) -> ("Image"=→"Collimation Image":T1, "Measure Report"=→"Measurement Report":string)
            }
            frame "Current Position[mm]" {
              n128 = call "Read Axis Position data.vi"("error in (no error)"=w255, "Fiber Auto Collimation state data in"=w254) -> ("error out"=w251:errorcluster, "Current position"=w253:dbl[unit])  [unwired: 7 in, 1 out]
              n129 = node(w253) -> (→"Current Position[mm]":dbl)
              n130 = call <userlib>:"Convert True to Enabled.vi"("Enable?"=TRUE) -> ("Enabled"=w249:T6)  [unwired: 2 in]
              n131 = property on="Up" class="Bool"("DisabledEnum"=w249) -> ()  [unwired: 2 in, 2 out]
              n132 = property on="Down" class="Bool"("DisabledEnum"=w249) -> ()  [unwired: 2 in, 2 out]
              n133 = property on="Home" class="Bool"("DisabledEnum"=w249) -> ()  [unwired: 2 in, 2 out]
            }
            frame "Monitored Watt indicator" {
              # "Errors shouldn't be a problem if the only trigger for this case is the Monitor event occuring.  \n\nIf other things can trigger this case, then some error clearning may need to be done here to prevent instrument class errors from being generated (for instance, if this control is updated before the instrument has been initialized)."
              # "The incoming state data isn't used in the example for anything, but it could be used for a real program (to determine things like appearance, visibility, etc.)"
              # "This example case doesn't use the \"State Data\" object to get the value because the value is the \"latest notification\" from the Watt Notifier reference.  \n\nThe \"latest notification\" is essentially a form of \"State Data\" because the code in the Model loop can get it at any time in exactly the same way as it's being obtained here."
              # "This should be the \"Obtain XXXX Notifier\" matching the type of Monitor in use.  Switch it to a different notifier obtainer if not Watts."
              # "This is the enum that should contain all of the station's instrument identifiers.  It should have the one that does the monitoring for this indicator selected."
              # "This case is just here as a demo of how a Monitor event would be used to change the appearance of an Indicator properly using the station template.  \n\nThis code either needs to be changed to match an actual Monitor being used, or deleted if no Monitor is being used or if the Monitor handling is done elsewhere.\n#ChangeThis"
              n134 = call <instrlib>:"Get instrument reference by identifier.vi"("error in (no error)"=w265, "Identifier"=Instrument_list."" ("Instrument list")) -> ("error out"=w263:errorcluster, "nLight Instrument.lvclass"=w262:refnum<class "nLight Instrument.lvclass">)  [unwired: 7 in, 1 out]
              n135 = call-dynamic "Obtain Monitor.vi"("error in (no error)"=w263, "nLight Instrument in"=w262) -> ("error out"=w261:errorcluster, "Monitor reference out"=w260:refnum<class "Monitor.lvclass">)  [unwired: 7 in, 1 out]
              n136 = call-dynamic "Obtain wattage notifier.vi"("error in (no error)"=w261, "Monitor in"=w260) -> ("error out"=w259:errorcluster, "Wattage notifier"=w258:refnum<notifier>)  [unwired: 7 in, 1 out]
              n137 = Get Notifier Status(notifier=w258, error in (no error)=w259) -> (current notification=→"Monitored Watt indicator":dbl[unit], error out=w256:errorcluster)  [unwired: 3 out]
            }
            frame "Station information" {
              w283 = FALSE ("Error on not found (T)")
              # "The \"software version\" field should be displayed somewhere in nearly all cases.  If it's removed from here, it needs to be made accessible elsewhere (for instance, in a \"Help->About\" menu option).\n\nThe other fields displayed in the default readout may be removed if considered unnecessary or confusing for a given station, or extra fields added.\n#CheckDefault"
              n138 = call <userlib>:"Look up string key.vi"("Error on not found (T)"=w283, "Key [string/enum]"=String_keys."Software name" ("Station config string keys"), "error in (no error)"=w269, "nLight Recipe in"=w268) -> ("error out"=w285:errorcluster, "String Key Value"=w287:string, "nLight Recipe out"=w286:refnum<class "Station config.lvclass">)  [unwired: 4 in, 1 out]
              n139 = call <userlib>:"Look up string key.vi"("Error on not found (T)"=w283, "Key [string/enum]"=String_keys."Software version" ("Station config string keys"), "error in (no error)"=w285, "nLight Recipe in"=w286) -> ("error out"=w280:errorcluster, "String Key Value"=w282:string, "nLight Recipe out"=w281:refnum<class "Station config.lvclass">)  [unwired: 4 in, 1 out]
              n140 = call <userlib>:"Read Site.vi"("error in (no error)"=w280, "Station config in"=w281) -> ("error out"=w278:errorcluster, "Site"=w270:T11, "Station config out"=w279:refnum<class "Station config.lvclass">)  [unwired: 7 in]
              n141 = call <userlib>:"Read Environment.vi"("error in (no error)"=w278, "Station config in"=w279) -> ("error out"=w276:errorcluster, "Environment"=w271:T12, "Station config out"=w277:refnum<class "Station config.lvclass">)  [unwired: 7 in]
              n142 = call-dynamic "Read Station number.vi"("error in (no error)"=w276, "Station config in"=w277) -> ("error out"=w274:errorcluster, "Station number"=w272:i32, "Station config out"=w275:refnum<class "Station config.lvclass">)  [unwired: 7 in]
              n143 = call <userlib>:"Read Equipment ID.vi"("error in (no error)"=w274, "Station config in"=w275) -> ("error out"=w266:errorcluster, "Equipment ID"=w273:string)  [unwired: 7 in, 1 out]
              n144 = Format Into String(format string="Software name: %s\nSoftware version: %s\nSite: %s\nEnvironment: %s\nNEQdb Station number: %d\nMOM Equipment ID: %s", w287, w282, w270, w271, w272, w273) -> (resulting string=→"Station information":string)  [unwired: 2 in, 1 out]
            }
          }
        }
        n145 = Bundle("事件注册引用句柄"=w193, "事件注册引用句柄"=w198) -> (w192:T7)  [unwired: 1 in]
        n146 = property class="Pnl"(reference=w187, error in=w183, "DeferPanUpdts"=FALSE ("Defer Panel Updates")) -> (error out=w177:errorcluster)  [unwired: 1 out]
        n147 = call <userlib>:"Trash error.vi"("error in"=w177) -> ()  [unwired: 15 in]
      }
    }
    n148 = call "Apex view loop error handler.vi"("errors in"=w70) -> ("error out"=w72:errorcluster)  [unwired: 10 in]
  }
  n149 = while {
    tunnel: [w295] -> w23
    tunnel: w50 -> [w294]
    tunnel: w5 -> [w291]
    tunnel: dbl[unit][] [0.005, 0.001, 9.999999999999999e-05, 4.9999999999999996e-05, 1.9999999999999998e-05, 9.999999999999999e-06] -> [w290]
    stop <- w293 stop-if-true
    # "For easy copying"
    # "Controller loop.  All \"value change\" events, and any triggered by user action (menus, keys, mouse clicks, etc.).  Most event states should do nothing except enqueue to the Model loop.\nValues from associated controls should be sent to the Model in the Variant data, so reading from local variables and property nodes is allowed.  Not allowed: writing to indicators, property nodes, local variables, or global variables.  No invoke nodes."
    n150 = event "Controller [Value change events go here]" shown="[5] \"Save Data\": 值改变" {
      selector: w294 -> [_ _ _ _ _ _ _ _ _ _ _ _ _ _ _ _ _ _ _ _ _ _ _]
      dyn-events: _ -> [_ _ _ _ _ _ _ _ _ _ _ _ _ _ _ _ _ _ _ _ _ _ _]
      timeout: _ -> [_ _ _ _ _ _ _ _ _ _ _ _ _ _ _ _ _ _ _ _ _ _ _]
      tunnel: [TRUE _ _ _ _ _ _ _ _ _ _ _ _ _ _ _ _ _ _ _ _ _ _] -> w293
      tunnel: [w296 w301 w310 w312 w313 w315 w317 w319 w323 w329 w335 _ _ _ _ w362 w367 w372 w377 w380 w383 w385 w388] -> w292
      tunnel: w291 -> [_ _ _ _ _ _ _ _ _ _ _ w341 _ _ _ _ _ _ _ _ _ _ _]
      tunnel: w290 -> [_ _ _ _ _ _ _ _ _ _ _ w339 _ _ _ _ _ _ _ _ _ _ _]
      event User Event {
        n151 = event-data() -> ()  [unwired: 1 in, 5 out]
        n152 = call <vilib>:"Clear Errors.vi"() -> ("error out"=w296:errorcluster)  [unwired: 6 in, 1 out]
      }
      event Panel Close? {
        # "If this was live LabVIEW, we always want the window to stay open. during runtime.\nIf this was an EXE, the window only closes after all the program is done, at which point the \"Exit\" call closes it.\nSo we always want to discard this here."
        # "If a \"Quit\" button or menu option is added in addition to this event (which fires when the \"X\" to close is clicked), then make sure both cases run the same code.\n\nIf there are conditions that should prevent the \"quit\" case from running (for instance, by default it's not allowed to quit during a test), instead of checking for them here or in the Model loop \"Quit\" case, it might be better to have the \"View\" loop set the \"FP.Closeable\" property of the main VI to False, and disabling any other menu item or button that also attempts to quit.  \n#CheckDefault"
        n153 = event-data() -> ()  [unwired: 1 in, 4 out]
        n154 = call "Software name constant.vi"() -> ("Software name constant"=w298:string)
        n155 = Format Into String(format string="Are you sure you want to exit %s?" ("message"), w298) -> (resulting string=w304:string)  [unwired: 2 in, 1 out]
        n156 = Two Button Dialog(message=w304, 1:"Cancel" ("F button name (\"Cancel\")"), 2:"Yes, exit" ("T button name (\"OK\")")) -> (T button?=w300:bool)
        n157 = case shown="真" w300 {
          tunnel: [_ w307] -> w301
          frame False {
          }
          frame True {
            n158 = call "Enqueue one state to model.vi"("Enqueued state"="Quit") -> ("error out"=w307:errorcluster)  [unwired: 10 in]
          }
        }
        n159 = event-data("Discard?"=TRUE) -> ()  [unwired: 1 in, 1 out]
      }
      event "Cancel Test": Value Change {
        # "This puts the \"Cancel Test\" ahead of any other state. \n\nProbably what should always happen, but be sure to be aware that the \"Cancel Test\" state will by default clear out all pending cases besides \"End Test\" that are enqueued, (to prevent any queued test states from resuming immediately after the Cancel Test state runs).\n#CheckDefault"
        n160 = event-data() -> ()  [unwired: 1 in, 6 out]
        n161 = call "Enqueue one state to model.vi"("Priority? (F)"=TRUE, "Enqueued state"="Cancel Test") -> ("error out"=w310:errorcluster)  [unwired: 9 in]
      }
      event "Start Test": Value Change {
        n162 = event-data() -> ()  [unwired: 1 in, 6 out]
        n163 = call "Enqueue one state to model.vi"("Enqueued state"="Start test") -> ("error out"=w312:errorcluster)  [unwired: 10 in]
      }
      event "Collimation": Value Change {
        n164 = event-data() -> ()  [unwired: 1 in, 6 out]
        n165 = call "Enqueue one state to model.vi"("Enqueued state"="Collimation") -> ("error out"=w313:errorcluster)  [unwired: 10 in]
      }
      event "Save Data": Value Change {
        n166 = event-data() -> ()  [unwired: 1 in, 6 out]
        n167 = call "Enqueue one state to model.vi"("Enqueued state"="Save Data") -> ("error out"=w315:errorcluster)  [unwired: 10 in]
      }
      event "Spot detection": Value Change {
        n168 = event-data() -> ()  [unwired: 1 in, 6 out]
        n169 = call "Enqueue one state to model.vi"("Enqueued state"="Signal Defect detection") -> ("error out"=w317:errorcluster)  [unwired: 10 in]
      }
      event "Defect detection": Value Change {
        n170 = event-data() -> ()  [unwired: 1 in, 6 out]
        n171 = call "Enqueue one state to model.vi"("Enqueued state"="Surface defect identify") -> ("error out"=w319:errorcluster)  [unwired: 10 in]
      }
      event "Home": Value Change {
        n172 = event-data() -> ()  [unwired: 1 in, 6 out]
        n173 = call <userlib>:"Convert True to Enabled.vi"("Enable?"=FALSE) -> ("Enabled"=w321:T6)  [unwired: 2 in]
        n174 = property on="Up" class="Bool"("DisabledEnum"=w321) -> ()  [unwired: 2 in, 2 out]
        n175 = property on="Down" class="Bool"("DisabledEnum"=w321) -> ()  [unwired: 2 in, 2 out]
        n176 = property on="Collimation" class="Bool"("DisabledEnum"=w321) -> ()  [unwired: 2 in, 2 out]
        n177 = property on="Start Test" class="Bool"("DisabledEnum"=w321) -> ()  [unwired: 2 in, 2 out]
        n178 = call "Enqueue one state to model.vi"("Enqueued state"="Home") -> ("error out"=w323:errorcluster)  [unwired: 10 in]
      }
      event "Up": Value Change {
        n179 = event-data() -> ()  [unwired: 1 in, 6 out]
        n180 = call <userlib>:"Convert True to Enabled.vi"("Enable?"=FALSE) -> ("Enabled"=w325:T6)  [unwired: 2 in]
        n181 = property on="Down" class="Bool"("DisabledEnum"=w325) -> ()  [unwired: 2 in, 2 out]
        n182 = property on="Home" class="Bool"("DisabledEnum"=w325) -> ()  [unwired: 2 in, 2 out]
        n183 = property on="Collimation" class="Bool"("DisabledEnum"=w325) -> ()  [unwired: 2 in, 2 out]
        n184 = property on="Start Test" class="Bool"("DisabledEnum"=w325) -> ()  [unwired: 2 in, 2 out]
        n185 = local read "Distance"() -> (w327:dbl[unit])
        n186 = To Variant(anything=w327) -> (Variant=w328:variant)
        n187 = call "Enqueue one state to model.vi"("Enqueued data"=w328, "Enqueued state"="Up") -> ("error out"=w329:errorcluster)  [unwired: 9 in]
      }
      event "Down": Value Change {
        n188 = event-data() -> ()  [unwired: 1 in, 6 out]
        n189 = call <userlib>:"Convert True to Enabled.vi"("Enable?"=FALSE) -> ("Enabled"=w331:T6)  [unwired: 2 in]
        n190 = property on="Up" class="Bool"("DisabledEnum"=w331) -> ()  [unwired: 2 in, 2 out]
        n191 = property on="Home" class="Bool"("DisabledEnum"=w331) -> ()  [unwired: 2 in, 2 out]
        n192 = property on="Collimation" class="Bool"("DisabledEnum"=w331) -> ()  [unwired: 2 in, 2 out]
        n193 = property on="Start Test" class="Bool"("DisabledEnum"=w331) -> ()  [unwired: 2 in, 2 out]
        n194 = local read "Distance"() -> (w334:dbl[unit])
        n195 = To Variant(anything=w334) -> (Variant=w333:variant)
        n196 = call "Enqueue one state to model.vi"("Enqueued data"=w333, "Enqueued state"="Down") -> ("error out"=w335:errorcluster)  [unwired: 9 in]
      }
      event "Step Size 1", "Step Size 2", "Step Size 3", "Step Size 4", "Step Size 5", "Step Size 6": Value Change {
        n197 = event-data() -> ("CtlRef"=w340:refnum<vi>)  [unwired: 1 in, 5 out]
        n198 = Search 1D Array(1D array=w341, element=w340) -> (index of element=w338:i32)  [unwired: 1 in]
        n199 = Index Array(array=w339, index=w338) -> (element=→"Distance":dbl[unit])
      }
      event "Manual Mode": Value Change {
        n200 = event-data() -> ("NewVal"=w342:bool)  [unwired: 1 in, 5 out]
        n201 = Not(x=w342) -> (.not. x?=w343:bool)
        n202 = call <userlib>:"Convert True to Enabled.vi"("Enable?"=w342) -> ("Enabled"=w345:T6)  [unwired: 2 in]
        n203 = call <userlib>:"Convert True to Enabled.vi"("Enable?"=w343) -> ("Enabled"=w344:T6)  [unwired: 2 in]
        n204 = property on="Collimation" class="Bool"("DisabledEnum"=w345) -> ()  [unwired: 2 in, 2 out]
        n205 = property on="Defect detection" class="Bool"("DisabledEnum"=w345) -> ()  [unwired: 2 in, 2 out]
        n206 = property on="Start Test" class="Bool"("DisabledEnum"=w344) -> ()  [unwired: 2 in, 2 out]
      }
      event "Auto Mode": Value Change {
        n207 = event-data() -> ("NewVal"=w347:bool)  [unwired: 1 in, 5 out]
        n208 = Not(x=w347) -> (.not. x?=w348:bool)
        n209 = call <userlib>:"Convert True to Enabled.vi"("Enable?"=w348) -> ("Enabled"=w349:T6)  [unwired: 2 in]
        n210 = call <userlib>:"Convert True to Enabled.vi"("Enable?"=w347) -> ("Enabled"=w346:T6)  [unwired: 2 in]
        n211 = property on="Collimation" class="Bool"("DisabledEnum"=w349) -> ()  [unwired: 2 in, 2 out]
        n212 = property on="Defect detection" class="Bool"("DisabledEnum"=w349) -> ()  [unwired: 2 in, 2 out]
        n213 = property on="Start Test" class="Bool"("DisabledEnum"=w346) -> ()  [unwired: 2 in, 2 out]
      }
      event "SN-1", "SN-2", "SN-3", "SN-4", "SN-5": Value Change {
        n214 = event-data() -> ()  [unwired: 1 in, 6 out]
        n215 = call <vilib>:"Trim Whitespace.vi"("string"="SN-1") -> ("trimmed string"=w358:string)  [unwired: 1 in]
        n216 = call <vilib>:"Trim Whitespace.vi"("string"="SN-2") -> ("trimmed string"=w356:string)  [unwired: 1 in]
        n217 = call <vilib>:"Trim Whitespace.vi"("string"="SN-3") -> ("trimmed string"=w353:string)  [unwired: 1 in]
        n218 = call <vilib>:"Trim Whitespace.vi"("string"="SN-4") -> ("trimmed string"=w352:string)  [unwired: 1 in]
        n219 = call <vilib>:"Trim Whitespace.vi"("string"="SN-5") -> ("trimmed string"=w351:string)  [unwired: 1 in]
        n220 = Build Array(w358, w356, w353, w352, w351) -> (w360:string[])
        n221 = property on="SN selection" class="CmbBox"("Value"=w358, "Strings[]"=w360) -> ()  [unwired: 2 in, 2 out]
      }
      event "SN selection": Value Change {
        n222 = event-data() -> ()  [unwired: 1 in, 6 out]
        n223 = To Variant(anything="SN selection") -> (Variant=w363:variant)
        n224 = call "Enqueue one state to model.vi"("Enqueued data"=w363, "Enqueued state"="Enter SN") -> ("error out"=w362:errorcluster)  [unwired: 9 in]
      }
      event "MOM Lot-2": Value Change {
        n225 = event-data() -> ()  [unwired: 1 in, 6 out]
        n226 = call <vilib>:"Trim Whitespace.vi"("string"="MOM Lot-2") -> ("trimmed string"=w365:string)  [unwired: 1 in]
        n227 = To Variant(anything=w365) -> (Variant=w368:variant)
        n228 = call "Enqueue one state to model.vi"("Enqueued data"=w368, "Enqueued state"="MOM Lot") -> ("error out"=w367:errorcluster)  [unwired: 9 in]
      }
      event "Fiber Ass PN": Value Change {
        n229 = event-data() -> ()  [unwired: 1 in, 6 out]
        n230 = call <vilib>:"Trim Whitespace.vi"("string"="Fiber Ass PN") -> ("trimmed string"=w371:string)  [unwired: 1 in]
        n231 = To Variant(anything=w371) -> (Variant=w373:variant)
        n232 = call "Enqueue one state to model.vi"("Enqueued data"=w373, "Enqueued state"="Enter Fiber Ass PN") -> ("error out"=w372:errorcluster)  [unwired: 9 in]
      }
      event "Operator": Value Change {
        n233 = event-data() -> ()  [unwired: 1 in, 6 out]
        n234 = call <vilib>:"Trim Whitespace.vi"("string"="Operator") -> ("trimmed string"=w376:string)  [unwired: 1 in]
        n235 = To Variant(anything=w376) -> (Variant=w378:variant)
        n236 = call "Enqueue one state to model.vi"("Enqueued data"=w378, "Enqueued state"="Enter Operator") -> ("error out"=w377:errorcluster)  [unwired: 9 in]
      }
      event "Enter MOM Lot": Value Change {
        n237 = event-data() -> ()  [unwired: 1 in, 6 out]
        n238 = call "Enqueue one state to model.vi"("Enqueued state"="Enter MOM Lot") -> ("error out"=w380:errorcluster)  [unwired: 10 in]
      }
      event "Remote stop config panel": Value Change {
        n239 = event-data() -> ()  [unwired: 1 in, 6 out]
        n240 = call "Enqueue one state to model.vi"("Enqueued state"="Close config panel") -> ("error out"=w383:errorcluster)  [unwired: 10 in]
      }
      event "Open and embed config panel": Value Change {
        n241 = event-data() -> ()  [unwired: 1 in, 6 out]
        n242 = control-ref of="Sub Panel example space"() -> (w384:refnum<vi>)
        n243 = call "Enqueue one state to model.vi"("Enqueued data"=w384, "Enqueued state"="Open config panel") -> ("error out"=w385:errorcluster)  [unwired: 9 in]
      }
      event "Open config panel": Value Change {
        n244 = event-data() -> ()  [unwired: 1 in, 6 out]
        n245 = call "Enqueue one state to model.vi"("Enqueued state"="Open config panel") -> ("error out"=w388:errorcluster)  [unwired: 10 in]
      }
    }
    n246 = disable-structure shown="Disabled" {
      frame Disabled {
        n247 = call "Enqueue one state to model.vi"() -> ()  [unwired: 11 in, 1 out]
      }
      frame Enabled {
      }
    }
    n248 = call "Apex controller loop error handler.vi"("error in"=w292) -> ("error out"=w295:errorcluster)  [unwired: 10 in]
  }
  n249 = control-ref of="This VI"() -> (w37:refnum<vi>)
  n250 = call "Emergency kill loop by reference.vi"("Quit early notifier"=w35, "VI reference in"=w37) -> ("error out"=w24:errorcluster)  [unwired: 9 in]
  n251 = call <vilib>:"Clear Errors.vi"("error in (no error)"=w31) -> ("error out"=w36:errorcluster)  [unwired: 5 in, 1 out]
  n252 = Send Notification(notification=TRUE, notifier=w35, error in (no error)=w36) -> (error out=w25:errorcluster)  [unwired: 1 out]
  n253 = call <userlib>:"Merge errors no loss micro.vi"("error in (no error) 1"=w31, "error in (no error) 5"=w25, "error in (no error) 6"=w23, "error in (no error) 7"=w24) -> ("error out"=w26:errorcluster)  [unwired: 5 in]
  n254 = call "Unregister panel from running.vi"("error in (no error)"=w26, "Fiber Auto Collimation panel in"=w14) -> ("error out"=→"error out":errorcluster, "Fiber Auto Collimation panel out"=→"Fiber Auto Collimation main panel out":refnum<class "Fiber Auto Collimation main panel.lvclass">)  [unwired: 8 in]
